vi "Generate Documentation--dialog.vi"(8 "error in":errorcluster, 11 "Project Path":path) -> (0 "error out":errorcluster)   [LabVIEW 2019, in "Panther Dashboard.lvlib"]
uses:
  Panther Dashboard.lvlib
  <vilib>/Wovalab/AntiDoc/Document Type/Add-ons/LabVIEW Project/Lv Proj/Lv Proj.lvclass
  C:/Program Files (x86)/National Instruments/LabVIEW 2019/vi.lib/Wovalab/AntiDoc/Document Type/Document/Document Type.lvclass
  <vilib>/Utility/miscctls.llb/LVPointTypeDef.ctl
  <vilib>/Wovalab/AntiDoc/Document Type/Add-ons/LabVIEW Project/Lv Proj Config/Lv Proj Config.lvclass
  C:/Program Files (x86)/National Instruments/LabVIEW 2019/vi.lib/Wovalab/AntiDoc/Document Type/Config/Config.lvclass
  <vilib>/Wovalab/AntiDoc/Document Type/Document/Document Type.lvclass/Document Type.ctl
  <vilib>/Wovalab/AntiDoc/Document Type/Add-ons/LabVIEW Project/Lv Proj Config/Lv Proj Config.lvclass/Lv Proj Config.ctl
  <vilib>/Wovalab/AntiDoc/Doc/Author Info--cluster.ctl
  <vilib>/Wovalab/AntiDoc/Doc/Doc.lvclass/Doc.ctl
  <vilib>/Wovalab/AntiDoc/Document Type/Document/Read Config.vi
  <vilib>/Wovalab/AntiDoc/Document Type/Add-ons/LabVIEW Project/Lv Proj Config/Write Project Path.vi
  <vilib>/Wovalab/AntiDoc/Document Type/Document/Write Config.vi
  <vilib>/Wovalab/AntiDoc/Doc/Write Document File Name.vi
  <vilib>/Wovalab/AntiDoc/Doc/Write Documentation Folder.vi
  <vilib>/Wovalab/AntiDoc/Document Type/Config/Config.lvclass
  <vilib>/Wovalab/AntiDoc/Progress Bar/Progress Bar.lvlib
  <vilib>/Wovalab/AntiDoc/Document Type/Document/Document Type.lvclass
  <vilib>/Wovalab/AntiDoc/Doc/Doc.lvclass
panel:
  in  "Open the document at the end of the generation":bool=TRUE
  in  "Generate":bool
  out "Progress Bar":u8(slide) caption="Waiting for user action..." max=100 scale=0.0..100.0
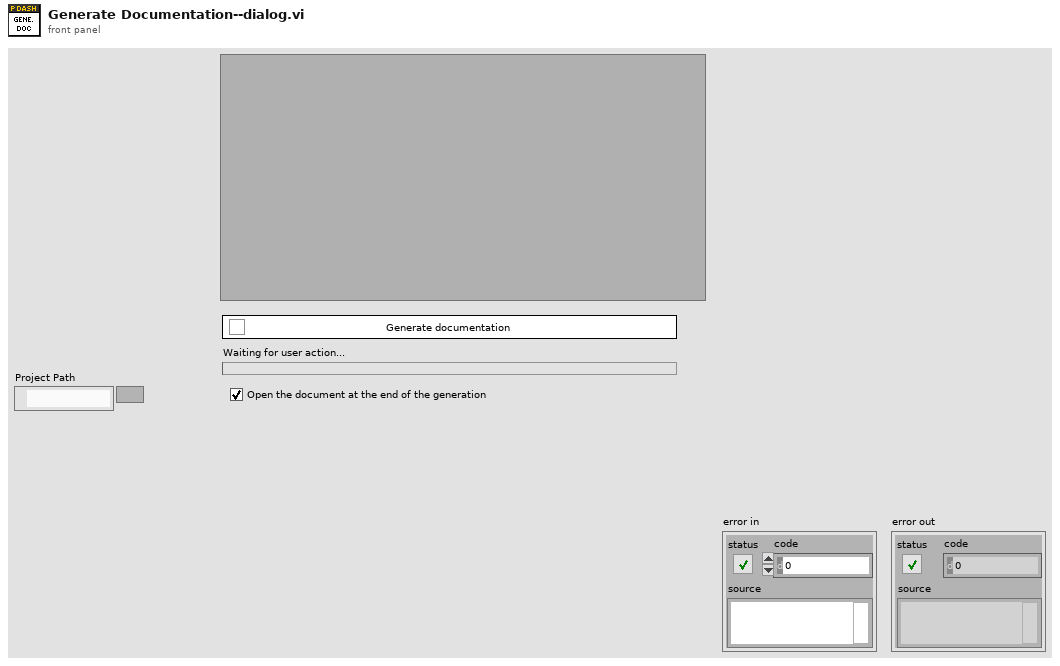
[diagram p1: front panel]
types:
  T1 = enum32{"Invalid", "Standard", "Closed", "Hidden", "Minimized", "Maximized"}
  T2 = typedef "LVPointTypeDef.ctl" = cluster{"Horizontal":i16, "Vertical":i16}
  T3 = typedef "AntiDoc.lvlib/Doc.lvclass/Author Info--cluster.ctl" = cluster{"Name":string, "Email":string}
  T4 = typedef "AntiDoc.lvlib/Document Type.lvclass/Final Documentation Info--cluster.ctl" = cluster{"Title":string, "Author Name":string, "Author Email":string, "Destination Folder":path, "File Name":string}
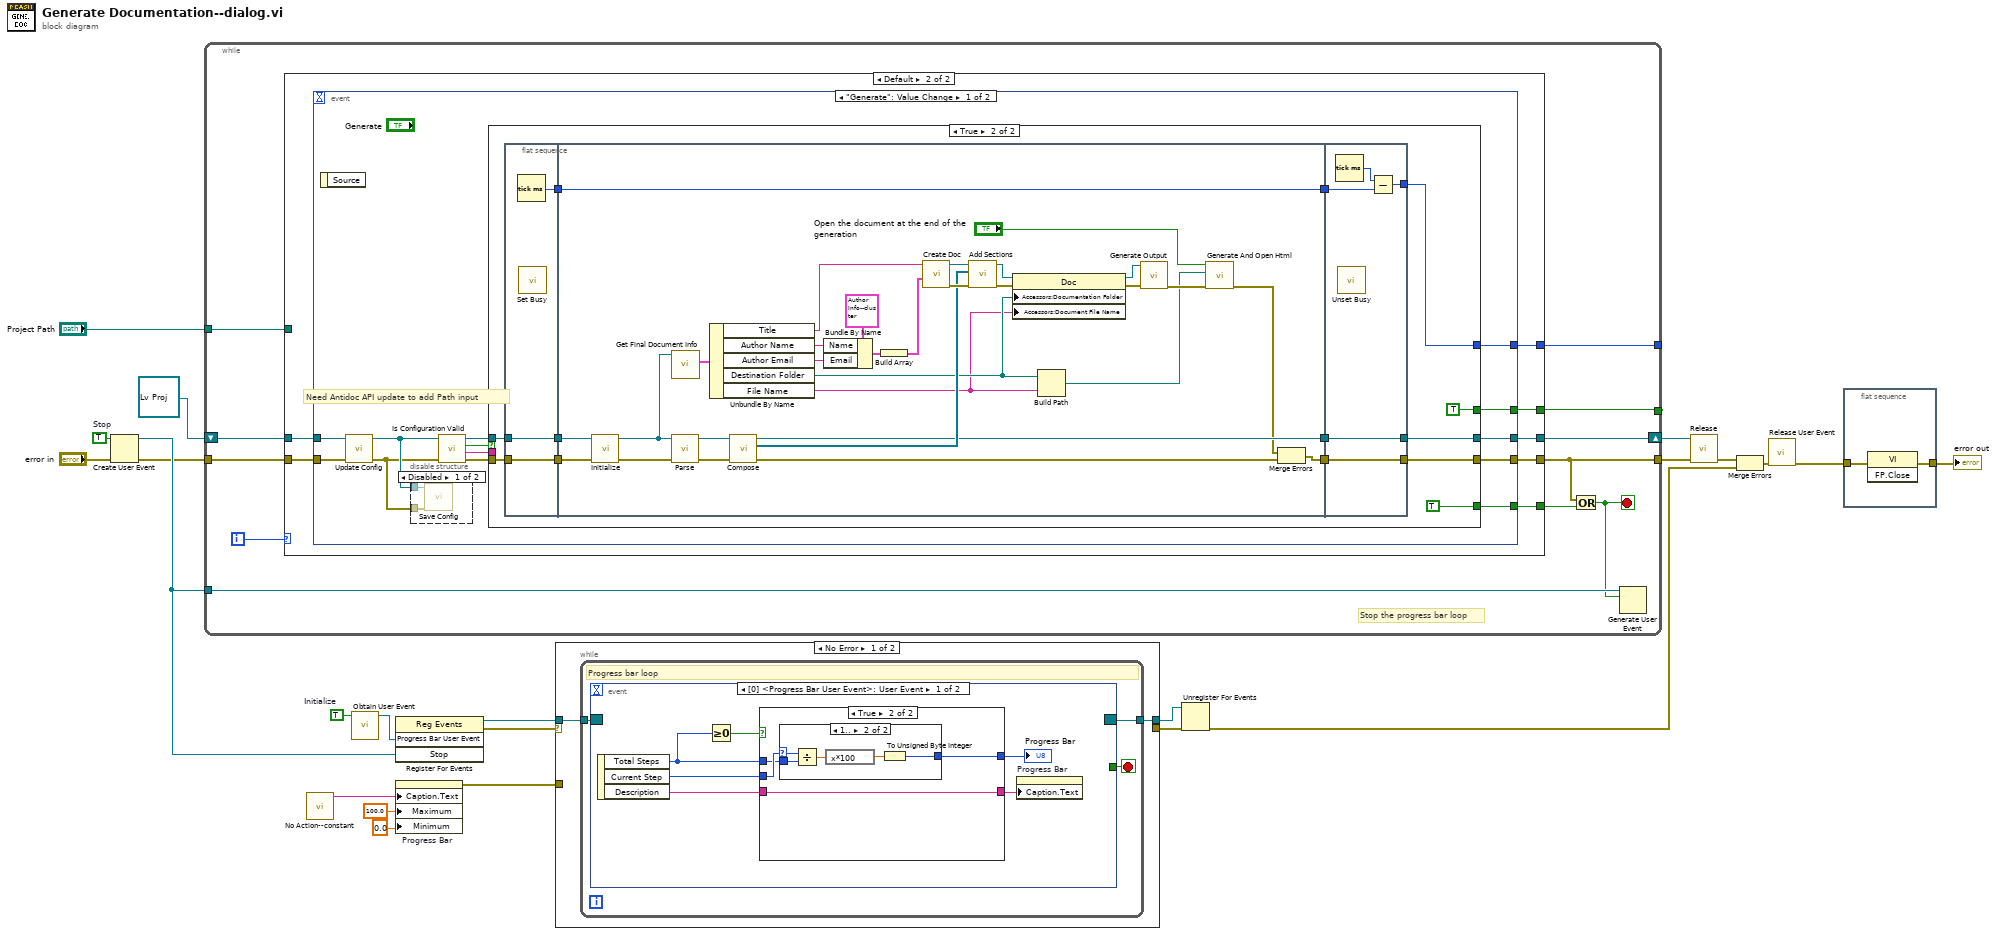
[diagram p0: block diagram]
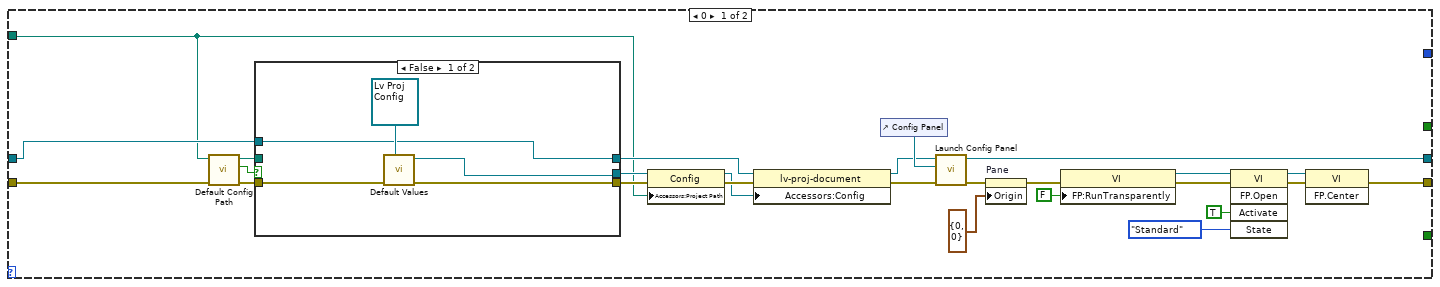
[diagram p2: hidden frame]
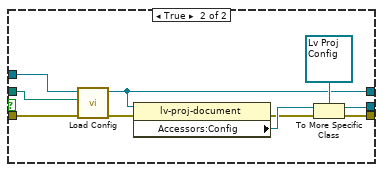
[diagram p3: hidden frame]
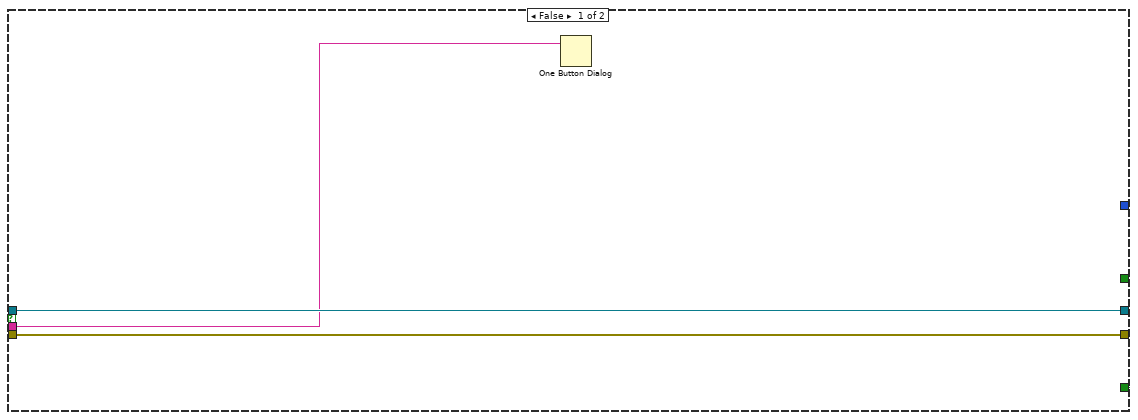
[diagram p5: hidden frame]
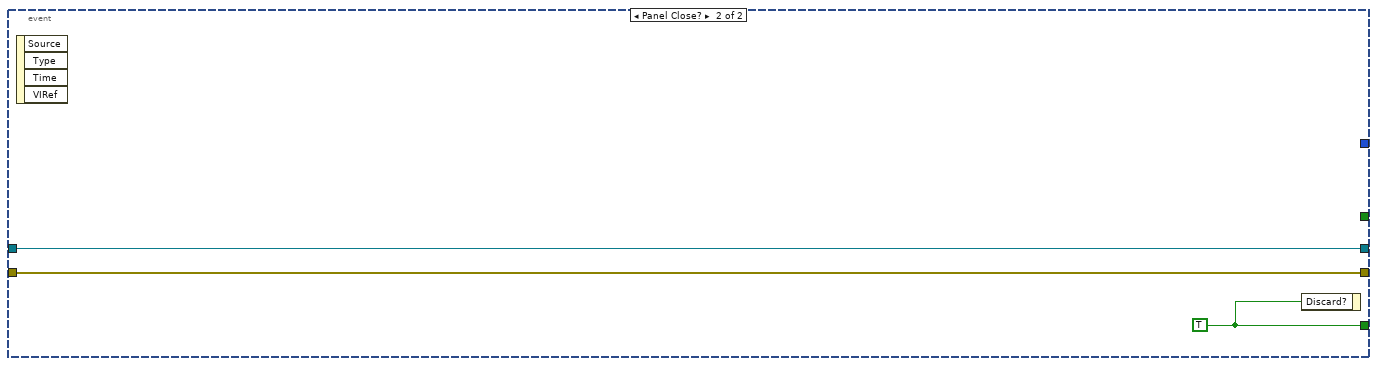
[diagram p6: hidden frame]
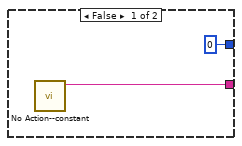
[diagram p7: hidden frame]
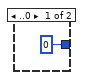
[diagram p8: hidden frame]
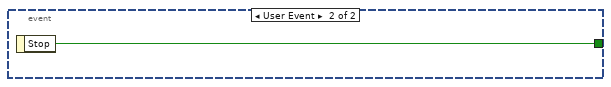
[diagram p9: hidden frame]
diagram:
  w13 = TRUE  # Initialize
  w23 = TRUE  # Stop
  n1 = Create User Event(user event datatype=w23, error in="error in") -> (user event=w12:refnum<user-event>, error out=w11:errorcluster)
  n2 = while {
    tunnel: [w27] -> w6
    tunnel: w12 -> [w34]
    tunnel: [w32] -> _
    tunnel: [w31] -> _
    shift-right: [w29] -> w7
    shift-left: refnum<class "Lv Proj.lvclass"> refnum ("Lv Proj Document Type.lvlib:lv-proj-document") -> [w33]
    tunnel: w11 -> [w28]
    tunnel: "Project Path" -> [w24]
    i -> [w30]
    stop <- w26 stop-if-true
    # "Stop the progress bar loop"
    n3 = case shown="Default" w30 {
      tunnel: [w54 w82] -> w27
      tunnel: [_ w81] -> w25
      tunnel: w33 -> [w40 w80]
      tunnel: [_ w79] -> w32
      tunnel: [w48 w78] -> w29
      tunnel: [_ w77] -> w31
      tunnel: w28 -> [w37 w76]
      tunnel: w24 -> [w39 _]
      frame 0 {
        n4 = call "Default Config Path.vi"("error in"=w37, "Project Path"=w39) -> ("error out"=w38:errorcluster, "File Exists?"=w36:bool, "Config Path"=w35:path)  [unwired: 7 in]
        n5 = case shown="False" w36 {
          tunnel: [w63 w74] -> w47
          tunnel: [w64 w71] -> w46
          tunnel: [w61 w69] -> w41
          tunnel: w40 -> [w61 w68]
          tunnel: w38 -> [w65 w67]
          tunnel: w35 -> [_ w66]
          frame False {
            n6 = call-dynamic "Default Values.vi"("Type"=refnum<class "Lv Proj Config.lvclass"> refnum ("Lv Proj Document Type.lvlib:Config"), "error in"=w65) -> ("error out"=w64:errorcluster, "Config out"=w63:refnum<class "Lv Proj Config.lvclass">)  [unwired: 8 in]
          }
          frame True {
            n7 = call <vilib>:"Load Config.vi"("error in"=w67, "File Path"=w66, "Document in"=w68) -> ("error out"=w70:errorcluster, "Document out"=w69:refnum<class "Lv Proj.lvclass">)  [unwired: 7 in]
            n8 = property class="lv-proj-document"(reference=w69, error in=w70) -> (error out=w72:errorcluster, "Accessors:Config"=w75:refnum<class "Config.lvclass">)  [unwired: 1 out]
            n9 = To More Specific Class(target class=refnum<class "Lv Proj Config.lvclass"> refnum ("Lv Proj Document Type.lvlib:Config"), reference=w75, error in=w72) -> (specific class reference=w74:refnum<class "Lv Proj Config.lvclass">, error out=w71:errorcluster)
          }
        }
        n10 = property class="Config"(reference=w47, error in=w46, "Accessors:Project Path"=w39) -> (reference out=w43:refnum<class "Lv Proj Config.lvclass">, error out=w45:errorcluster)
        n11 = property class="lv-proj-document"(reference=w41, error in=w45, "Accessors:Config"=w43) -> (reference out=w42:refnum<class "Lv Proj.lvclass">, error out=w44:errorcluster)
        n12 = control-ref of="Config Panel"() -> (w49:refnum<vi>)
        n13 = call <vilib>:"Launch Config Panel.vi"("error in"=w44, "Sub Panel"=w49, "Document in"=w42) -> ("error out"=w59:errorcluster, "Document out"=w48:refnum<class "Lv Proj.lvclass">)  [unwired: 7 in]
        n14 = property on="Pane" class="Pane"(error in=w59, "Origin"=T2 {"Horizontal"=0, "Vertical"=0}) -> (error out=w53:errorcluster)  [unwired: 1 in, 1 out]
        n15 = property class="VI"(error in=w53, "FP:RunTransparently"=FALSE ("Front Panel Window:Run VI Transparently")) -> (reference out=w50:refnum<vi>, error out=w52:errorcluster)  [unwired: 1 in]
        n16 = invoke class="VI" method="FP.Open"(reference=w50, error in=w52, "Activate"=TRUE ("Activate?"), "State"=T1."Standard") -> (reference out=w57:refnum<vi>, error out=w58:errorcluster)  [unwired: 1 in, 3 out]
        n17 = invoke class="VI" method="FP.Center"(reference=w57, error in=w58) -> (error out=w54:errorcluster)  [unwired: 1 in, 2 out]
      }
      frame Default {
        n18 = event shown="[0] \"Generate\": Value Change" {
          selector: _ -> [_ _]
          dyn-events: _ -> [_ _]
          timeout: _ -> [_ _]
          tunnel: [w95 w153] -> w82
          tunnel: [w94 w155] -> w81
          tunnel: w80 -> [w90 w154]
          tunnel: [w92 _] -> w79
          tunnel: [w91 w154] -> w78
          tunnel: [w89 _] -> w77
          tunnel: w76 -> [w87 w153]
          event "Generate": Value Change {
            # "Need Antidoc API update to add Path input"
            n19 = event-data() -> ()  [unwired: 1 in, 1 out]
            n20 = call <vilib>:"Update Config.vi"("error in"=w87, "Document in"=w90) -> ("error out"=w83:errorcluster, "Document out"=w84:refnum<class "Lv Proj.lvclass">)  [unwired: 8 in]
            n21 = disable-structure shown="Disabled" {
              disable-tunnel: w84 -> [w97 _]
              disable-tunnel: w83 -> [w96 _]
              frame Disabled {
                n22 = call <vilib>:"Save Config.vi"("error in"=w96, "Document in"=w97) -> ()  [unwired: 9 in, 1 out]
              }
              frame Enabled {
              }
            }
            n23 = call-dynamic "Is Configuration Valid.vi"("error in"=w83, "Document in"=w84) -> ("error out"=w86:errorcluster, "Details"=w88:string, "Valid?"=w93:bool, "Document out"=w85:refnum<class "Lv Proj.lvclass">)  [unwired: 6 in]
            n24 = case shown="True" w93 {
              tunnel: [w98 w113] -> w95
              tunnel: [FALSE TRUE ("event data")] -> w94
              tunnel: w85 -> [w100 w108]
              tunnel: [_ w107] -> w92
              tunnel: [w100 w103] -> w91
              tunnel: [_ TRUE] -> w89
              tunnel: w88 -> [w99 _]
              tunnel: w86 -> [w98 w104]
              frame False {
                n25 = One Button Dialog(message=w99) -> ()  [unwired: 1 in, 1 out]
              }
              frame True {
                n26 = flat-sequence {
                  tunnel: [w117] -> w110
                  tunnel: [w116] -> w109
                  tunnel: w108 -> [w116]
                  tunnel: [w115] -> w105
                  tunnel: w104 -> [w115]
                  tunnel: [w133] -> w114
                  tunnel: [w138] -> w111
                  tunnel: w110 -> [w138]
                  tunnel: w109 -> [w134]
                  tunnel: w105 -> [w132]
                  tunnel: [w122] -> w102
                  tunnel: [w152] -> w113
                  tunnel: w114 -> [w152]
                  tunnel: w111 -> [w150]
                  tunnel: [w149] -> w107
                  tunnel: [w148] -> w103
                  tunnel: w102 -> [w148]
                  frame #0 {
                    n27 = Tick Count (ms)() -> (millisecond timer value=w117:u32)
                    n28 = call <vilib>:"Set Busy.vi"() -> ()  [unwired: 10 in, 2 out]
                  }
                  frame #1 {
                    n29 = call-dynamic "Initialize.vi"("error in"=w132, "Document in"=w134) -> ("error out"=w131:errorcluster, "Document out"=w130:refnum<class "Lv Proj.lvclass">)  [unwired: 8 in]
                    n30 = call-dynamic "Parse.vi"("error in"=w131, "Document in"=w130) -> ("error out"=w136:errorcluster, "Document out"=w137:refnum<class "Lv Proj.lvclass">)  [unwired: 8 in]
                    n31 = call-dynamic "Get Final Document Info.vi"("Document in"=w130) -> ("Final Documentation Info"=w129:T4)  [unwired: 9 in, 1 out]
                    n32 = Unbundle By Name(w129) -> ("Title"=w128:string, "Author Name"=w127:string, "Author Email"=w126:string, "Destination Folder"=w125:path, "File Name"=w124:string)
                    n33 = call-dynamic "Compose.vi"("error in"=w136, "Document in"=w137) -> ("error out"=w123:errorcluster, "Sections"=w135:refnum<class "Section.lvclass">[], "Document out"=w122:refnum<class "Lv Proj.lvclass">)  [unwired: 7 in]
                    n34 = Bundle By Name(cluster=T3 {"Name"="Wovalab", "Email"="contact@wovalab.com"} ("Author Info"), "Name"=w127, "Email"=w126) -> (w140:T3)
                    n35 = Build Array(w140) -> (w139:T3[])
                    n36 = call <vilib>:"Create Doc.vi"("Authors"=w139, "Title"=w128) -> ("error out"=w147:errorcluster, "Doc out"=w144:refnum<class "Doc.lvclass">)  [unwired: 8 in]
                    n37 = call <vilib>:"Add Sections.vi"("error in (no error)"=w147, "Sections"=w135, "Doc in"=w144) -> ("error out"=w146:errorcluster, "Doc out"=w143:refnum<class "Doc.lvclass">)  [unwired: 7 in]
                    n38 = property class="Doc"(reference=w143, error in=w146, "Accessors:Documentation Folder"=w125, "Accessors:Document File Name"=w124) -> (reference out=w142:refnum<class "Doc.lvclass">, error out=w145:errorcluster)
                    n39 = Build Path(base path=w125, name or relative path=w124) -> (appended path=w119:path)
                    n40 = call <vilib>:"Generate Output.vi"("error in"=w145, "Doc in"=w142) -> ("error out"=w121:errorcluster)  [unwired: 8 in, 1 out]
                    n41 = call "Generate And Open Html.vi"("error in"=w121, "Generated File Path"=w119, "Open Generated Document"="Open the document at the end of the generation") -> ("error out"=w120:errorcluster)  [unwired: 8 in]
                    n42 = Merge Errors(w120, w123) -> (w133:errorcluster)
                  }
                  frame #2 {
                    n43 = Tick Count (ms)() -> (millisecond timer value=w151:u32)
                    n44 = call <vilib>:"Unset Busy.vi"() -> ()  [unwired: 11 in, 1 out]
                    n45 = Subtract(x=w151, y=w150) -> (x-y=w149:u32)
                  }
                }
              }
            }
          }
          event Panel Close? {
            w155 = TRUE
            n46 = event-data() -> ()  [unwired: 1 in, 4 out]
            n47 = event-data("Discard?"=w155) -> ()  [unwired: 1 in, 1 out]
          }
        }
      }
    }
    n48 = Or(x=w27, y=w25) -> (x .or. y?=w26:bool)
    n49 = Generate User Event(user event=w34, event data cluster=w26) -> ()  [unwired: 2 in, 2 out]
  }
  n50 = call <vilib>:"No Action--constant.vi"() -> ("No Action"=w20:string)  [unwired: 11 in]
  n51 = call <vilib>:"Obtain User Event.vi"("Initialize(F)"=w13) -> ("Progress Bar User Event"=w14:refnum<user-event>)  [unwired: 10 in]
  n52 = register-events(w14, w12) -> (reference out=w15:refnum<event-registration>, error out=w16:errorcluster)  [unwired: 2 in]
  n53 = property on="Progress Bar" class="Slide (strict)"("Caption.Text"=w20, "Maximum"=100.0 ("Data Entry Limits:Maximum"), "Minimum"=0.0 ("Data Entry Limits:Minimum")) -> (error out=w19:errorcluster)  [unwired: 2 in, 1 out]
  n54 = case shown="No Error" w16 {
    selector: w16 -> [_ w180]
    tunnel: w15 -> [w157 w181]
    tunnel: [w156 w181] -> w17
    tunnel: [_ w180] -> w18
    tunnel: w19 -> [_ _]
    frame No Error {
      n55 = while {
        tunnel: w157 -> [w160]
        tunnel: [w158] -> w156
        stop <- w159 stop-if-true
        # "Progress bar loop"
        n56 = event shown="[0] <Progress Bar User Event>: User Event" {
          selector: w160 -> [_ _]
          dyn-events: [_ _] -> w158
          timeout: _ -> [_ _]
          tunnel: [_ w179] -> w159
          event User Event {
            n57 = event-data() -> ("Total Steps"=w163:i32, "Current Step"=w164:i32, "Description"=w165:string)  [unwired: 1 in]
            n58 = Greater Or Equal To 0?(x=w163) -> (x >= 0?=w166:bool)
            n59 = case shown="True" w166 {
              tunnel: w165 -> [_ w169]
              tunnel: w164 -> [_ w172]
              tunnel: w163 -> [_ w171]
              tunnel: [u8 0 w170] -> w162
              tunnel: [w168 w169] -> w161
              frame False {
                n60 = call <vilib>:"No Action--constant.vi"() -> ("No Action"=w168:string)  [unwired: 11 in]
              }
              frame True {
                n61 = case shown="1.." w172 {
                  selector: w172 -> [_ w178]
                  tunnel: w171 -> [_ w177]
                  tunnel: [u8 0 w174] -> w170
                  frame ..0 {
                  }
                  frame 1.. {
                    n62 = Divide(x=w178, y=w177) -> (x/y=w175:dbl)
                    n63 = expression code="x*100"(w175) -> (w176:dbl)
                    n64 = To Unsigned Byte Integer(number=w176) -> (unsigned 8bit integer=w174:u8)
                  }
                }
              }
            }
            "Progress Bar" <- w162
            n65 = property on="Progress Bar" class="Slide (strict)"("Caption.Text"=w161) -> ()  [unwired: 2 in, 2 out]
          }
          event User Event {
            n66 = event-data() -> ("Stop"=w179:bool)  [unwired: 1 in]
          }
        }
      }
    }
    frame Error {
    }
  }
  n67 = Unregister For Events(event registration refnum=w17, error in=w18) -> (error out=w9:errorcluster)
  n68 = call-dynamic "Release.vi"("error in"=w6, "Document in"=w7) -> ("error out"=w5:errorcluster)  [unwired: 9 in]
  n69 = Merge Errors(w5, w9) -> (w8:errorcluster)
  n70 = call <vilib>:"Release User Event.vi"("error in"=w8) -> ("error out"=w3:errorcluster)  [unwired: 10 in]
  n71 = flat-sequence {
    tunnel: w3 -> [w183]
    tunnel: [w182] -> w2
    frame #0 {
      n72 = invoke class="VI" method="FP.Close"(error in=w183) -> (error out=w182:errorcluster)  [unwired: 2 in, 2 out]
    }
  }
  "error out" <- w2
